vi "Subvi FIFO OUT.vi"(0 "FIFOOUTenable":bool, 3 "FIFOOUT":refnum<k21>="FIFOOUTa", 4 "number 8":u8, 5 "number 1":u8, 6 "number 7":u8, 7 "number 2":u8, 8 "number 6":u8, 9 "number 5":u8, 10 "number 4":u8, 11 "number 3":u8) -> (1 "FIFOOUT mon":bool)   [LabVIEW 2017]
uses:
  GV FIFOOUT gate.vi
  GV gated pixelclock change.vi
  <vilib>/rvi/DataTransferAndStorage/Container/Common/niFpgaContainerExecOnDevCompGetState.vi
  <vilib>/rvi/Emulation/niFpgaEmulationIsFPGAContextNoSignature.vi
  <vilib>/rvi/Emulation/niFpgaSctlEmulationGetInTimedLoop.vi
  <vilib>/rvi/errors/niFpgaSetErrorForExecOnDevCompSimple.vi
  <vilib>/rvi/eio/common/nirviEmuReportErrorAndStop.vi
  <vilib>/rvi/DataTransferAndStorage/Container/Common/niFpgaContainerGetUniqueNameForEmu.vi
  <vilib>/rvi/FIFO/Fifo_Resource/nirvififoEmulationSetSize.vi
  <vilib>/rvi/FIFO/Fifo_Resource/nirviFifoEmulationQueueMgr.vi
  <instcachedir>/0/nirviFifoEmulationQueueMgr_E5CAEC123FF24DC58D834DCA3CDAA9B5.lvgen/nirviFifoEmulationQueueMgr_E5CAEC123FF24DC58D834DCA3CDAA9B5_001.vi
  <vilib>/rvi/FIFO/Fifo_Resource/nirvififoEmulationDetermineInputValidOut.vi
  <vilib>/rvi/FIFO/Fifo_Resource/nirvififoEmulationCreateLock.vi
  <vilib>/rvi/Emulation/niFpgaProcessEmulError.vi
  <vilib>/rvi/FIFO/Fifo_Resource/nirvififoEmulationObtainLock.vi
  <vilib>/rvi/FIFO/Fifo_Resource/nirvififoEmulationReleaseLock.vi
  <vilib>/rvi/occurrence/nirviWaitOnOccurrenceBase.vi
  <vilib>/rvi/errors/nirviReportUnexpectedCaseInternalError.vi
  <vilib>/rvi/errors/nirviReportUnexpectedCaseInternalError (U32).vi
  <vilib>/Utility/error.llb/Clear Errors.vi
  <vilib>/rvi/interface/RandomDataEmulation/niFpgaRandomDataHandleErrors.vi
  <vilib>/rvi/DataTransferAndStorage/Container/XNode/niFpgaContainer.xnode
  <vilib>/rvi/FIFO/Fifo_Resource/niFpgaFifoEmulationRefIn.vi
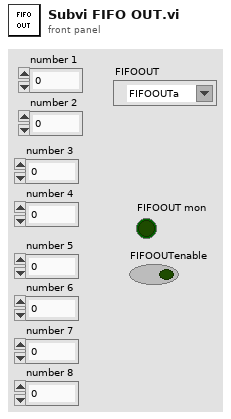
[diagram p1: front panel]
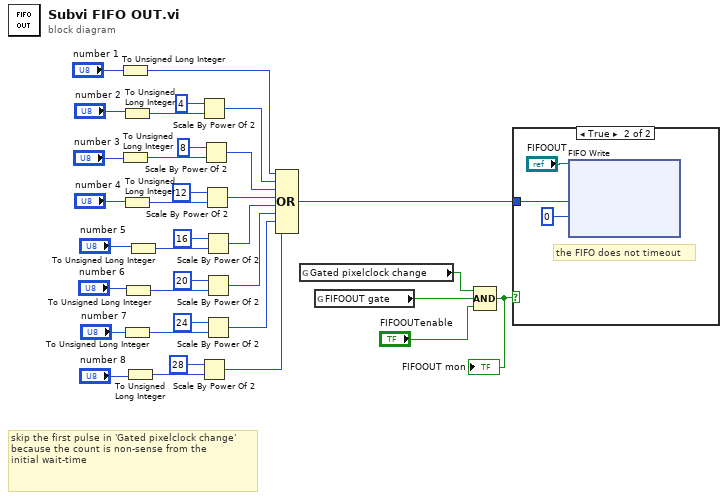
[diagram p0: block diagram]
diagram:
  # "skip the first pulse in 'Gated pixelclock change'\nbecause the count is non-sense from the\ninitial wait-time"
  n1 = To Unsigned Long Integer(number="number 1") -> (unsigned 32bit integer=w21:u32)
  n2 = To Unsigned Long Integer(number="number 3") -> (unsigned 32bit integer=w19:u32)
  n3 = To Unsigned Long Integer(number="number 2") -> (unsigned 32bit integer=w20:u32)
  n4 = To Unsigned Long Integer(number="number 4") -> (unsigned 32bit integer=w18:u32)
  n5 = To Unsigned Long Integer(number="number 7") -> (unsigned 32bit integer=w15:u32)
  n6 = To Unsigned Long Integer(number="number 6") -> (unsigned 32bit integer=w16:u32)
  n7 = To Unsigned Long Integer(number="number 8") -> (unsigned 32bit integer=w14:u32)
  n8 = To Unsigned Long Integer(number="number 5") -> (unsigned 32bit integer=w17:u32)
  n9 = Scale By Power Of 2(n=i16 4, x=w20) -> (x*2^n=w28:u32)
  n10 = Scale By Power Of 2(n=i16 28, x=w14) -> (x*2^n=w22:u32)
  n11 = Scale By Power Of 2(n=i16 8, x=w19) -> (x*2^n=w27:u32)
  n12 = Scale By Power Of 2(n=i16 12, x=w18) -> (x*2^n=w26:u32)
  n13 = Scale By Power Of 2(n=i16 16, x=w17) -> (x*2^n=w25:u32)
  n14 = Scale By Power Of 2(n=i16 20, x=w16) -> (x*2^n=w24:u32)
  n15 = Scale By Power Of 2(n=i16 24, x=w15) -> (x*2^n=w23:u32)
  n16 = Compound Arithmetic op=OR(w21, w28, w27, w26, w25, w24, w23, w22) -> (w4:u32)
  n17 = global read "GV gated pixelclock change.vi" "Gated pixelclock change"() -> (w5:bool)
  n18 = global read "GV FIFOOUT gate.vi" "FIFOOUT gate"() -> (w3:bool)
  n19 = Compound Arithmetic op=AND(w5, w3, "FIFOOUTenable") -> (w2:bool)
  "FIFOOUT mon" <- w2
  n20 = case shown="True" w2 {
    tunnel: w4 -> [_ w37]
    frame False {
    }
    frame True {
      # "the FIFO does not timeout"
      n21 = xnode ("FIFO Write")("Element"=w37, "Timeout"=0, "FIFO In"="FIFOOUT") -> ()  [unwired: 2 out]
    }
  }
